vi "Get Alias.vi"(8 "error in (no error)":errorcluster, 11 "Request Data in":refnum<class "Request Data.lvclass">) -> (0 "error out":errorcluster, 2 "Alias":string, 3 "Request Data out":refnum<class "Request Data.lvclass">)   [LabVIEW 2020, in "Publisher.lvlib" / "Request Data.lvclass"]
doc: "Return the Alias of the Data class.\nThe default implmentation returns the base class name."
uses:
  Request Data.lvclass
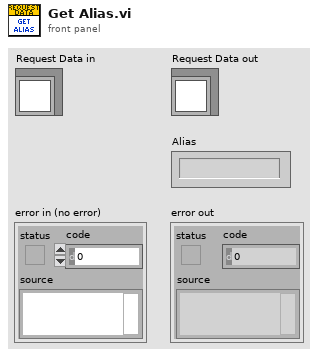
[diagram p1: front panel]
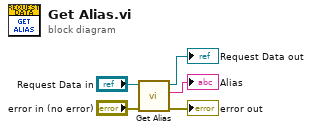
[diagram p0: block diagram]
diagram:
  n1 = call-dynamic "Get Alias.vi"("error in (no error)"="error in (no error)", "Request Data in"="Request Data in") -> ("error out"=→"error out":errorcluster, "Alias"=→"Alias":string, "Request Data out"=→"Request Data out":refnum<class "Request Data.lvclass">)  [unwired: 7 in]
